vi "Plot Initialize.vi"(5 "Plot Legend Color":u32(colorbox), 6 "Control Ref Cluster":T1, 7 "Main Frame Color":u32(colorbox), 8 "error in (no error)":errorcluster, 11 "2D Plot.lvclass in":refnum<class "2D Plot.lvclass">) -> (0 "error out":errorcluster, 3 "2D Plot.lvclass out":refnum<class "2D Plot.lvclass">)   [LabVIEW 2017, in "2D Plot.lvclass"]
uses:
  <vilib>/Math Plots/2D Math Plots/2D Plot/2D Plot/2D Plot.lvclass
  <vilib>/Math Plots/2D Math Plots/2D Plot/Action String/2DMathPlot Ctrl Act Cluster.ctl
  <vilib>/Math Plots/2D Math Plots/2D Plot/Action String/2DMathPlot State Class.ctl
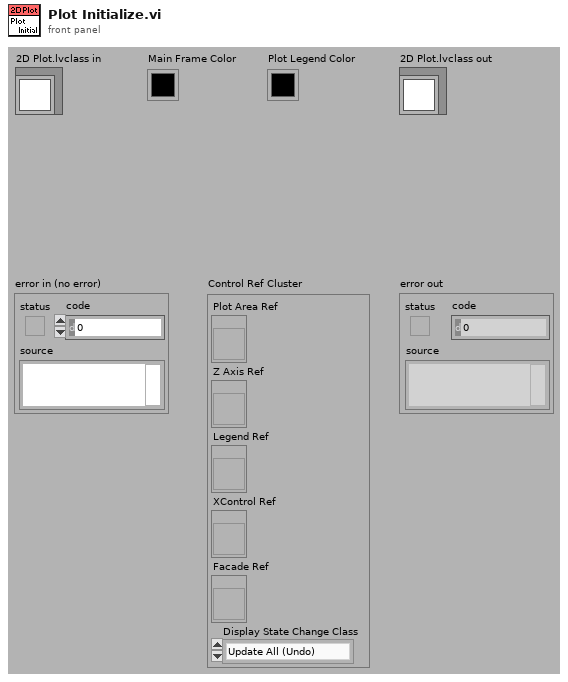
[diagram p1: front panel]
types:
  T1 = typedef "2DMathPlot Ctrl Act Cluster.ctl" = cluster{"Plot Area Ref":refnum<vi>, "Z Axis Ref":refnum<vi>, "Legend Ref":refnum<vi>, "XControl Ref":refnum<vi>, "Facade Ref":refnum<vi>, "Display State Change Class":T2}
  T2 = typedef "2DMathPlot State Class.ctl" = enum16{"Update All (Undo)", "Update General", "Update Appearance", "Update Format", "Update Scale", "Update Marker", "Update Cursor", "None"}
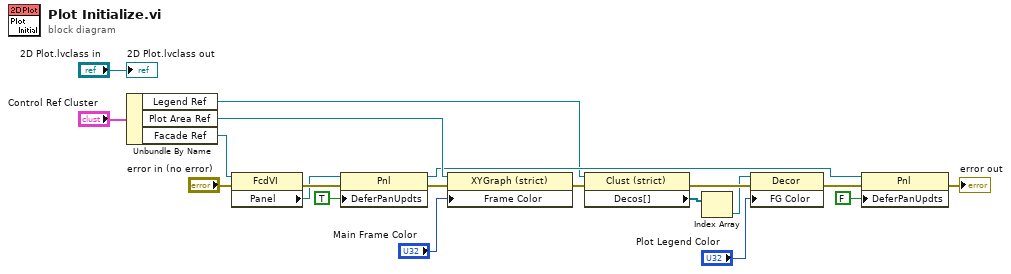
[diagram p0: block diagram]
diagram:
  n1 = Unbundle By Name("Control Ref Cluster") -> ("Legend Ref"=w7:refnum<vi>, "Plot Area Ref"=w15:refnum<vi>, "Facade Ref"=w13:refnum<vi>)
  n2 = property class="FcdVI"(reference=w13, error in="error in (no error)") -> (error out=w18:errorcluster, "Panel"=w16:refnum<vi>)  [unwired: 1 out]
  n3 = property class="Pnl"(reference=w16, error in=w18, "DeferPanUpdts"=TRUE ("Defer Panel Updates")) -> (reference out=w11:refnum<vi>, error out=w4:errorcluster)
  n4 = property class="XYGraph (strict)"(reference=w15, error in=w4, "Frame Color"="Main Frame Color") -> (error out=w3:errorcluster)  [unwired: 1 out]
  n5 = property class="Clust (strict)"(reference=w7, error in=w3) -> (error out=w10:errorcluster, "Decos[]"=w8:refnum<vi>[])  [unwired: 1 out]
  n6 = Index Array(array=w8) -> (element=w9:refnum<vi>)  [unwired: 1 in]
  n7 = property class="Decor"(reference=w9, error in=w10, "FG Color"="Plot Legend Color") -> (error out=w2:errorcluster)  [unwired: 1 out]
  n8 = property class="Pnl"(reference=w11, error in=w2, "DeferPanUpdts"=FALSE ("Defer Panel Updates")) -> (error out=→"error out":errorcluster)  [unwired: 1 out]
  "2D Plot.lvclass out" <- "2D Plot.lvclass in"
